vi "Set DDS Burst Delay Ns.vi"(8 "error in (no error)":errorcluster, 10 "ns":u64, 11 "channel_index":u8) -> (0 "error out":errorcluster)   [LabVIEW 2021, in "vmmso.lvlib"]
doc: "DLL_API void WINAPI SetDDSBurstDelayNs(unsigned char channel_index, unsigned long long int ns);"
uses:
  vmmso.lvlib
  vmmso.dll
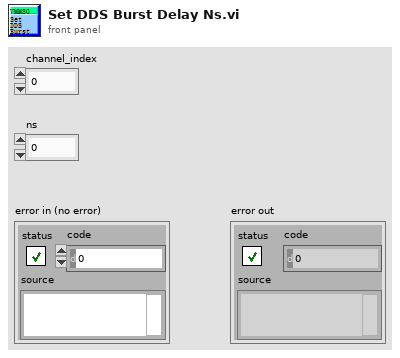
[diagram p1: front panel]
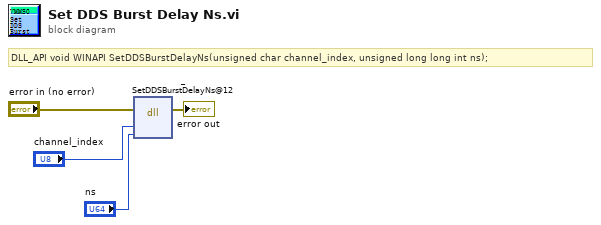
[diagram p0: block diagram]
diagram:
  # "DLL_API void WINAPI SetDDSBurstDelayNs(unsigned char channel_index, unsigned long long int ns);"
  n1 = dll-call lib="O:/MSO/library/demo-Labview/vmmso/vmmso.*" fn="_SetDDSBurstDelayNs@12"(error in="error in (no error)", "channel_index"="channel_index", "ns"="ns") -> (error out=→"error out":errorcluster)  [unwired: 5 in, 1 out]
